vi "Enable GUI Objects inside SomeTemplatesFound Tab.vi"(8 "error in":errorcluster, 11 "GUI Objects":T1) -> (0 "error out":errorcluster)   [LabVIEW 2020]
doc: "Enables all the GUI objects found inside the \"SomeTemplatesFound\" page of the Tab Control."
uses:
  GUI Objects.ctl
panel:
  # "Development\ncontrols/indicators useful for development and testing, but which are not outputs of the VI"
  # "Input\nInputs to the VI"
  # "Output\nOutputs of the VI"
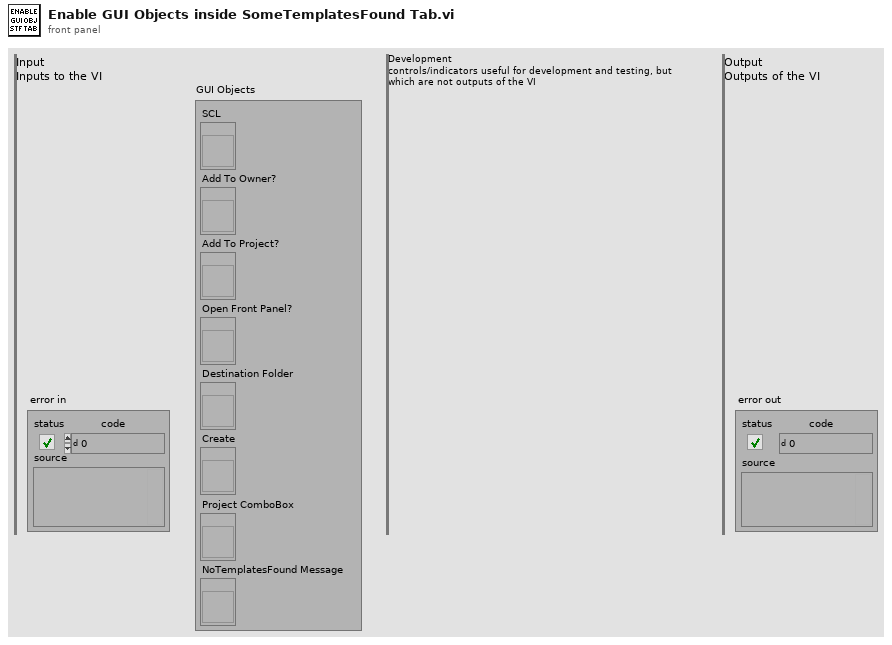
[diagram p1: front panel]
types:
  T1 = typedef "GUI Objects.ctl" = cluster{"SCL":refnum<vi>, "Add To Owner?":refnum<vi>, "Add To Project?":refnum<vi>, "Open Front Panel?":refnum<vi>, "Destination Folder":refnum<vi>, "Create":refnum<vi>, "Project ComboBox":refnum<vi>, "NoTemplatesFound Message":refnum<vi>}
  T2 = enum8{"Enabled", "Disabled", "Disabled and Grayed Out"}
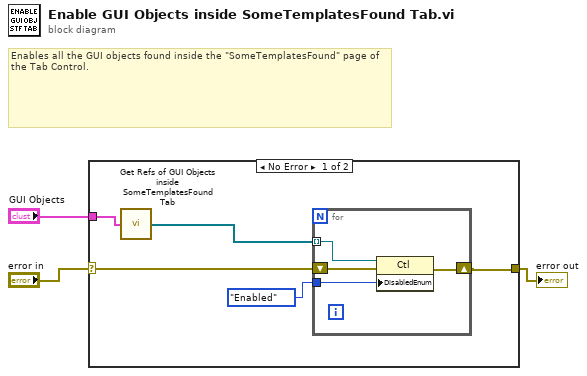
[diagram p0: block diagram]
diagram:
  # "Enables all the GUI objects found inside the \"SomeTemplatesFound\" page of the Tab Control."
  n1 = case shown="No Error" "error in" {
    selector: "error in" -> [w7 w13]
    tunnel: [w4 w13] -> w2
    tunnel: "GUI Objects" -> [w8 _]
    frame No Error {
      n2 = call "Get Refs of GUI Objects inside SomeTemplatesFound Tab.vi"("GUI Objects"=w8) -> ("Refs of GUI Objects inside SomeTemplatesFound Tab"=w6:refnum<vi>[])
      n3 = for {
        shift-right: [w11] -> w4
        shift-left: w7 -> [w12]
        tunnel: w6 -> [w10] mode=indexing
        tunnel: T2."Enabled" ("Disabled") -> [w9]
        n4 = property class="Ctl"(reference=w10, error in=w12, "DisabledEnum"=w9) -> (error out=w11:errorcluster)  [unwired: 1 out]
      }
    }
    frame Error {
    }
  }
  "error out" <- w2
